vi "FRC Color Processing Example.vi"() -> ()   [LabVIEW 2014]
uses:
  <vilib>/Rock Robotics/WPI/Camera/WPI_CameraSettings Read MJPG.ctl
  <vilib>/Rock Robotics/WPI/Camera/WPI_CameraImageSize.ctl
  Vision Support Code/Camera Types.ctl
  <vilib>/vision/NI_Vision_Development_Module.lvlib
panel:
  in  "Limit Tests?":bool=TRUE
  in  "Camera Type":T1=enum."MS HD3000 square"
  in  "Image Path":path=path "Sample Images/KicoffFilmingVision"
  in  "image files":string[](array[string])
  in  "Aspect Fudge Factor":dbl=1.0
  out "Detected Totes":T2(array[cluster]) {"Normalized Rect"."Numeric 5" format="%#_2g"; "Normalized Rect"."Numeric 3" format="%#_2g"; "Normalized Rect"."Numeric 2" format="%#_2g"; "Normalized Rect"."Numeric" format="%#_2g"}
  in  "Score Threshold":dbl=75.0
  in  "Show Carpet Mask":bool=TRUE
  in  "Source":enum32{"Files", "Camera"}(tab)
  in  "Images":i32(listbox)
  in  "Folder Location":path=path "C:/snobotics/LabView/Vision Images/Sample Images"
  in  "Camera Settings":T3={"fps"=20, "compression"=30, "Image Size"=enum."320x240"}
  in  "Camera Address":string="10.9.81.21"
  in  "Carpet Color":T5(tab)
  in  "Red":T6={"Hue"={231.0, 14.0}, "Sat"={83.0, 255.0}, "Val"={52.5, 255.0}} {"Hue" scale=0.0..255.0 scale format="%#_3g"}
  in  "Blue":T6={"Hue"={119.0, 181.0}, "Sat"={33.0, 255.0}, "Val"={48.571428571428584, 255.0}} {"Hue" scale=0.0..255.0 scale format="%#_3g"}
  in  "Annotate":bool=TRUE
  out "ms to process":u32
  out "Sorted Scores":T7(array[cluster]) {"Carpet" format="%#_3g"; "S" format="%#_3g"; "Trapezoid %" format="%#_3g"; "L" format="%#_3g"; "Area to CH" format="%#_3g"; "X" format="%#_3g"; "Y" format="%#_3g"}
  out "Particles":i32
  in  "Tote Color":T6={"Hue"={23.67058792990901, 48.923317529462665}, "Sat"={66.78571428571429, 255.0}, "Val"={48.571428571428584, 255.0}} {"Hue" scale=0.0..255.0 scale format="%#_3g"}
  out "Masked":T8(plugin-control)
  out "Original Image":T8(plugin-control)
  # "Instructions:\nUse Source to select image files from a directory or use a USB or IP camera connected to your laptop.\nUse Tote Color to threshold and build particles. Adjust calibration if needed.\nSelect which carpet color to use for scoring. Calibrate the colors if needed.\nAnnotations show the rectangle and the scores from top to bottom."
  # "Aspect Ratio"
  # "Density Profile"
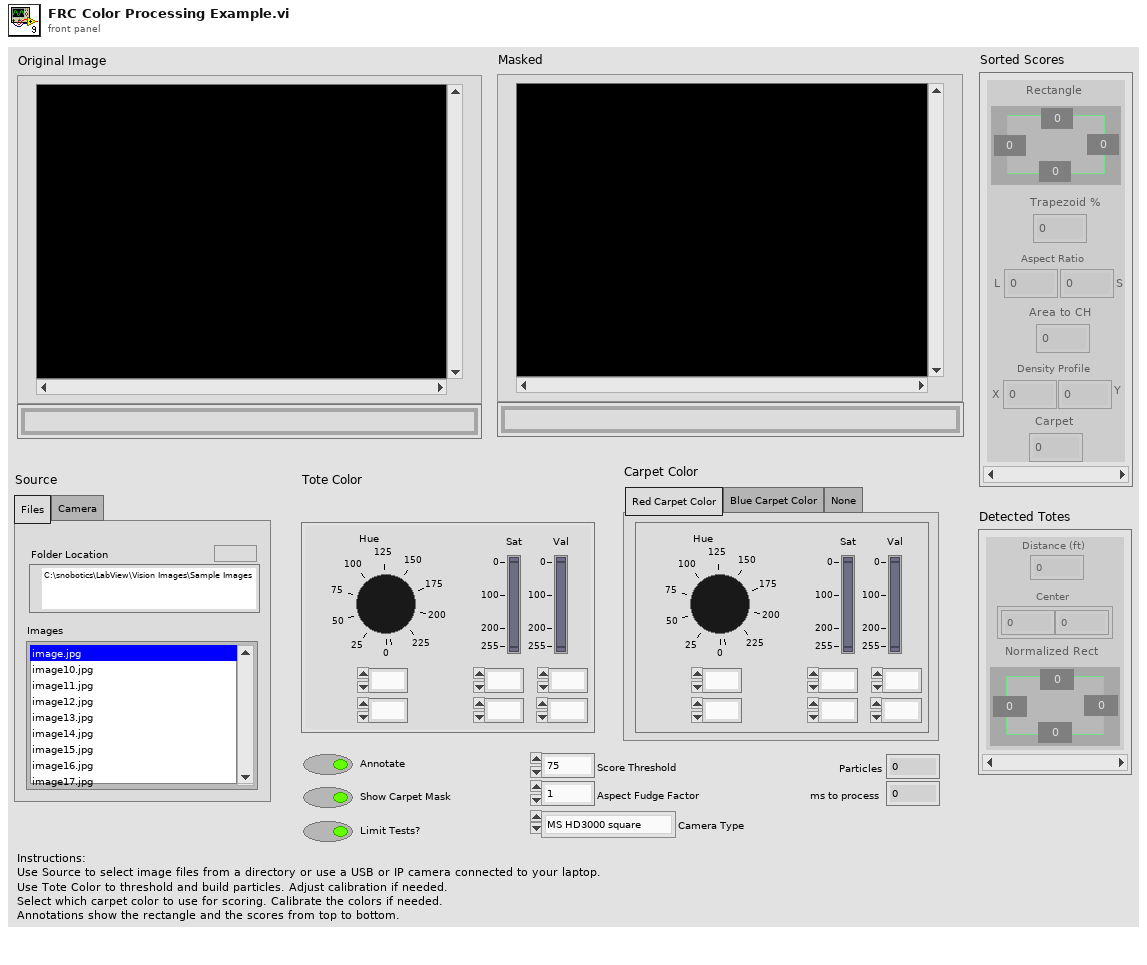
[diagram p1: front panel]
types:
  T1 = typedef "Camera Types.ctl" = enum16{"206", "1011", "1013", "MS HD3000 square", "MS HD3000 640x480"}
  T2 = cluster{"Distance (ft)":dbl, "Center":cluster{dbl, dbl}, "Normalized Rect":cluster{"Numeric":dbl, "Numeric 2":dbl, "Numeric 3":dbl, "Numeric 5":dbl}}[]
  T3 = typedef "WPI_CameraSettings Read MJPG.ctl" = cluster{"fps":i32, "compression":i32, "Image Size":T4}
  T4 = typedef "WPI_CameraImageSize.ctl" = enum16{"640x480", "320x240", "160x120", "Custom"}
  T5 = enum32{"Red Carpet Color", "Blue Carpet Color", "None"}
  T6 = cluster{"Hue":cluster{dbl, dbl}, "Sat":cluster{dbl, dbl}, "Val":cluster{dbl, dbl}}
  T7 = cluster{"Rectangle":cluster{"Numeric":dbl, "Numeric 2":dbl, "Numeric 3":dbl, "Numeric 5":dbl}, "Trapezoid %":dbl, "L":dbl, "S":dbl, "Area to CH":dbl, "X":dbl, "Y":dbl, "Carpet":dbl}[]
  T8 = typedef "IMAQ Image.ctl" = refnum<image>
  T9 = typedef "Particle Parameters" = i32
  T10 = typedef "Image Type" = u32
  T11 = cluster{"Bounding box":cluster{"left":dbl, "top":dbl, "right":dbl, "bottom":dbl}, "Trapezoid":dbl, "Long Aspect":dbl, "Short Aspect":dbl, "Area to CH":dbl, "X Mask":dbl, "Y Mask":dbl, "Carpet":dbl}[]
  T12 = cluster{"Red":cluster{"Hue":cluster{dbl, dbl}, "Sat":cluster{dbl, dbl}, "Val":cluster{dbl, dbl}}, "Blue":cluster{"Hue":cluster{dbl, dbl}, "Sat":cluster{dbl, dbl}, "Val":cluster{dbl, dbl}}}
  T13 = cluster{cluster{"[0]":dbl, "[1]":dbl, "[2]":dbl, "[3]":dbl}, "Score":dbl, "Long Edge Score":dbl, "Short Edge Score":dbl, dbl, "X Score":dbl, "Y Score":dbl, "Carpet":dbl}[]
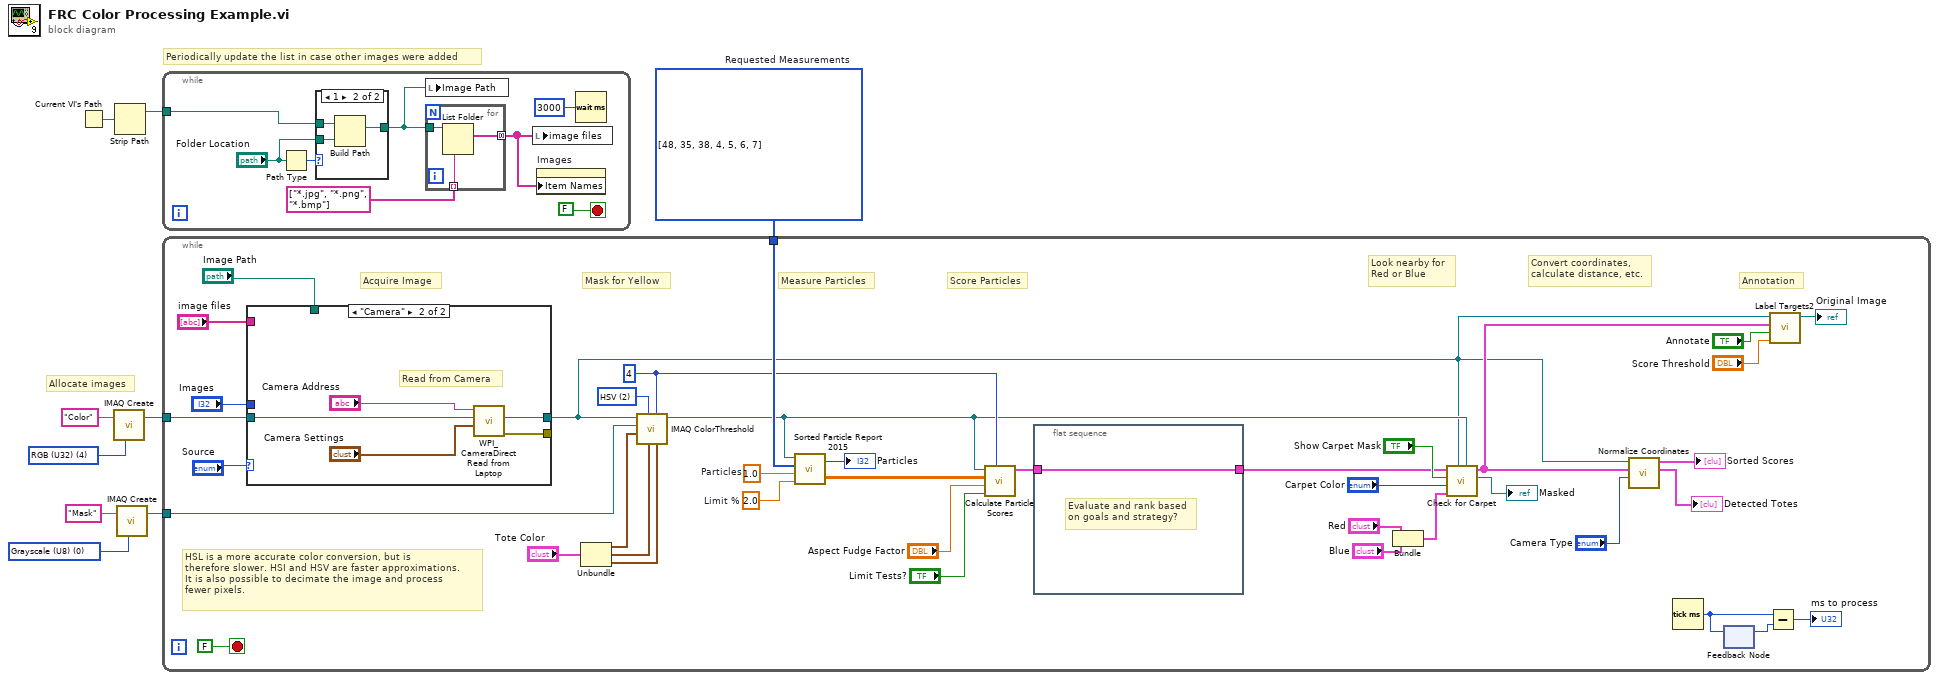
[diagram p0: block diagram]
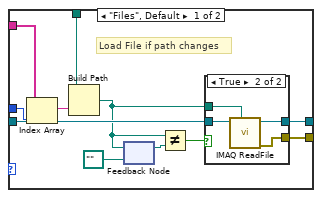
[diagram p3: hidden frame]
diagram:
  w3 = T9[] [48, 35, 38, 4, 5, 6, 7] items=["Center of Mass X", "Center of Mass Y", "First Pixel X", "First Pixel Y", "Bounding Rect Left", "Bounding Rect Top", "Bounding Rect Right", "Bounding Rect Bottom", "Max Feret Diameter Start X", "Max Feret Diameter Start Y", "Max Feret Diameter End X", "Max Feret Diameter End Y", "Max Horiz. Segment Length Left", "Max Horiz. Segment Length Right", "Max Horiz. Segment Length Row", "-", "Bounding Rect Width", "Bounding Rect Height", "Bounding Rect Diagonal", "Perimeter", "Convex Hull Perimeter", "Holes' Perimeter", "Max Feret Diameter", "Equivalent Ellipse Major Axis", "Equivalent Ellipse Minor Axis", "Equivalent Ellipse Minor Axis (Feret)", "Equivalent Rect Long Side", "Equivalent Rect Short Side", "Equivalent Rect Diagonal", "Equivalent Rect Short Side (Feret)", "Average Horiz. Segment Length", "Average Vert. Segment Length", "Hydraulic Radius", "Waddel Disk Diameter", "-", "Area", "Holes' Area", "Particle & Holes' Area", "Convex Hull Area", "Image Area", "-", "Number of Holes", "Number of Horiz. Segments", "Number of Vert. Segments", "-", "Orientation", "Max Feret Diameter Orientation", "-", "% Area/Image Area", "% Area/(Particle & Holes' Area)", "Ratio of Equivalent Ellipse Axes", "Ratio of Equivalent Rect Sides", "-", "Elongation Factor", "Compactness Factor", "Heywood Circularity Factor", "Type Factor", "-", "Sum X", "Sum Y", "Sum XX", "Sum XY", "Sum YY", "Sum XXX", "Sum XXY", "Sum XYY", "Sum YYY", "-", "Moment of Inertia XX", "Moment of Inertia XY", "Moment of Inertia YY", "Moment of Inertia XXX", "Moment of Inertia XXY", "Moment of Inertia XYY", "Moment of Inertia YYY", "Norm. Moment of Inertia XX", "Norm. Moment of Inertia XY", "Norm. Moment of Inertia YY", "Norm. Moment of Inertia XXX", "Norm. Moment of Inertia XXY", "Norm. Moment of Inertia XYY", "Norm. Moment of Inertia YYY", "Hu Moment 1", "Hu Moment 2", "Hu Moment 3", "Hu Moment 4", "Hu Moment 5", "Hu Moment 6", "Hu Moment 7"]  # Requested Measurements
  w6 = T10 0 items=["Grayscale (U8)", "Grayscale (I16)", "Grayscale (SGL)", "Complex (CSG)", "RGB (U32)", "HSL (U32)", "RGB (U64)", "Grayscale (U16)"] ("Image Type")
  w8 = T10 4 items=["Grayscale (U8)", "Grayscale (I16)", "Grayscale (SGL)", "Complex (CSG)", "RGB (U32)", "HSL (U32)", "RGB (U64)", "Grayscale (U16)"] ("Image Type")
  # "Periodically update the list in case other images were added"
  # "Allocate images"
  n1 = Current VI's Path() -> (path=w2:path)
  n2 = call "IMAQ Create"("Image Name"="Color", "Image Type"=w8) -> ("New Image"=w7:T8)  [unwired: 2 in, 2 out]
  n3 = Strip Path(path=w2) -> (stripped path=w1:path)  [unwired: 1 out]
  n4 = call "IMAQ Create"("Image Name"="Mask", "Image Type"=w6) -> ("New Image"=w4:T8)  [unwired: 2 in, 2 out]
  n5 = while {
    tunnel: w1 -> [w11]
    stop <- FALSE stop-if-true
    n6 = Path Type(1:"Folder Location") -> (0:w13:i16)
    n7 = case shown="1" w13 {
      tunnel: "Folder Location" -> [w18 w21]
      tunnel: [w18 w19] -> w10
      tunnel: w11 -> [_ w20]
      frame 0, Default {
      }
      frame 1 {
        n8 = Build Path(base path=w20, name or relative path=w21) -> (appended path=w19:path)
      }
    }
    n9 = local write "Image Path"(w10) -> ()
    n10 = for {
      tunnel: [w24] -> w14 mode=concatenating
      tunnel: w10 -> [w23]
      tunnel: string[] ["*.jpg", "*.png", "*.bmp"] -> [w22] mode=indexing
      n11 = List Folder(path=w23, pattern=w22) -> (filenames=w24:string[])  [unwired: 2 in, 3 out]
    }
    n12 = local write "image files"(w14) -> ()
    n13 = property on="Images" class="LstBox (strict)"("Item Names"=w14) -> ()  [unwired: 2 in, 2 out]
    n14 = Wait (ms)(milliseconds to wait=u32 3000) -> ()  [unwired: 1 out]
  }
  n15 = while {
    tunnel: w7 -> [w63]
    tunnel: w4 -> [w61]
    tunnel: w3 -> [w55]
    stop <- FALSE stop-if-true
    w38 = 4 ("Replace Value")
    w51 = 2.0  # Limit %
    w54 = 1.0  # Particles
    w60 = u16 2 items=["RGB", "HSL", "HSV", "HSI"] ("Color Mode")
    # "Measure Particles"
    # "Convert coordinates,\ncalculate distance, etc."
    # "Annotation"
    # "Score Particles"
    # "Mask for Yellow"
    # "Acquire Image"
    # "HSL is a more accurate color conversion, but is\ntherefore slower. HSI and HSV are faster approximations.\nIt is also possible to decimate the image and process\nfewer pixels."
    # "Look nearby for\nRed or Blue"
    n16 = case shown="\"Camera\"" "Source" {
      tunnel: [w75 w86] -> _
      tunnel: [w76 w85] -> w28
      tunnel: w63 -> [w74 w84]
      tunnel: "image files" -> [w66 _]
      tunnel: "Images" -> [w73 _]
      tunnel: "Image Path" -> [w71 _]
      frame "Files", Default {
        # "Load File if path changes"
        n17 = Index Array(array=w66, index=w73) -> (element=w72:string)
        n18 = Build Path(base path=w71, name or relative path=w72) -> (appended path=w67:path)
        n19 = feedback-in #1(w67) -> ()
        n20 = feedback #1(path "" ("appended path")) -> (w69:path)
        n21 = Not Equal?(x=w67, y=w69) -> (x != y?=w70:bool)
        n22 = case shown="True" w70 {
          tunnel: [w77 w81] -> w76
          tunnel: [_ w80] -> w75
          tunnel: w74 -> [w77 w79]
          tunnel: w67 -> [_ w78]
          frame False {
          }
          frame True {
            n23 = call "IMAQ ReadFile"("File Path"=w78, "Image"=w79) -> ("error out"=w80:errorcluster, "Image Out"=w81:T8)  [unwired: 5 in, 3 out]
          }
        }
      }
      frame "Camera" {
        # "Read from Camera"
        n24 = call <vilib>:"WPI_CameraDirect Read from Laptop.vi"("Camera Settings"="Camera Settings", "Image"=w84, "address"="Camera Address") -> ("error out"=w86:errorcluster, "Image Out"=w85:T8)  [unwired: 7 in]
      }
    }
    n25 = Unbundle("Tote Color") -> ("Hue"=w59:cluster{dbl, dbl}, "Sat"=w58:cluster{dbl, dbl}, "Val"=w57:cluster{dbl, dbl})
    n26 = call "IMAQ ColorThreshold"("Blue or Luma or Val or Inten Range"=w57, "Replace Value"=w38, "Green or Sat Range"=w58, "Color Mode"=w60, "Red or Hue Range"=w59, "Image Dst"=w61, "Image Src"=w28) -> ("Image Dst Out"=w29:T8)  [unwired: 3 in, 1 out]
    n27 = call "Sorted Particle Report 2015.vi"("Min Area Size %"=w51, "Particle Count Limit"=w54, "Pixel Measurements"=w55, "Image in"=w29) -> ("Sorted Data"=w52:dbl[][], "Particles"=→"Particles":i32)
    n28 = call "Calculate Particle Scores.vi"("Pixel Value"=w38, "Limit Tests?"="Limit Tests?", "Aspect Fudge Factor"="Aspect Fudge Factor", "Sorted Data"=w52, "Image in"=w29) -> ("Scores"=w31:T11)  [unwired: 6 in]
    n29 = flat-sequence {
      tunnel: w31 -> [w65]
      tunnel: [w65] -> w30
      frame #0 {
        # "Evaluate and rank based\non goals and strategy?"
      }
    }
    n30 = Bundle("Red"="Red", "Blue"="Blue") -> (w39:T12)  [unwired: 1 in]
    n31 = call "Check for Carpet.vi"("Original Mask"=w29, "Original Color"=w28, "Carpet Colors"=w39, "Carpet Selector"="Carpet Color", "Combine Carpet Mask"="Show Carpet Mask", "Initial Scores"=w30) -> ("Updated Mask"=→"Masked":T8, "Updated Scores"=w37:T13)  [unwired: 4 in]
    n32 = call "Normalize Coordinates.vi"("Camera Type"="Camera Type", "Targets"=w37, "Image in"=w28) -> ("Found Totes"=→"Detected Totes":T2, "Sorted Scores"=→"Sorted Scores":T7)  [unwired: 7 in]
    n33 = Tick Count (ms)() -> (millisecond timer value=w49:u32)
    n34 = feedback-in #2(w49) -> ()
    n35 = feedback #2() -> (w50:u32)  [unwired: 1 in]
    n36 = Subtract(x=w49, y=w50) -> (x-y=→"ms to process":u32)
    n37 = call "Label Targets2.vi"("Score Threshold"="Score Threshold", "Annotate"="Annotate", "Targets"=w37, "Image in"=w28) -> ("Image out"=→"Original Image":T8)  [unwired: 7 in]
  }
